vi "Initialize Attributes.vi"(8 "error in (no error)":errorcluster, 10 "Attribute Data":variant, 11 "CS++SimMotor in":refnum<class "CS++SimMotor.lvclass">) -> (0 "error out":errorcluster, 2 "Found?":bool, 3 "CS++SimMotor out":refnum<class "CS++SimMotor.lvclass">)   [LabVIEW 2015, in "CS++SimMotor.lvlib" / "CS++SimMotor.lvclass"]
doc: "Initialize object attribute.\n\nUnique resources should be allocated elsewhere!"
uses:
  CS++SimMotor.lvclass
  CSPP_Core/Classes/CS++ProcessVariables/ProcessVariable/PV.lvclass
  CSPP_Core/Actors/CS++BaseActor/CS++BaseActor.lvclass/CS++BaseActor.ctl
  CSPP_Core/Classes/CS++ProcessVariables/ProcessVariable/PV.lvclass/PV.ctl
  CS++SimMotor.lvclass/CS++SimMotor.ctl
  CSPP_Core/Classes/CS++ProcessVariables/ProcessVariable/Write PV URL.vi
  CSPP_Core/Classes/CS++ProcessVariables/ProcessVariable/Write Type Descriptor.vi
  <vilib>/Utility/error.llb/Error Cluster From Error Code.vi
  CSPP_DeviceBase/CS++Motor/CS++Motor.lvclass
  CSPP_Core/Classes/CS++BaseClasses/Factory/CS++Factory.lvclass
  CSPP_Core/Libraries/Utilities/CS++Utilities.lvlib
  CSPP_Core/Classes/CS++ProcessVariables/CS++ProcessVariables.lvlib
  CSPP_Core/Actors/CS++BaseActor/CS++BaseActor.lvclass
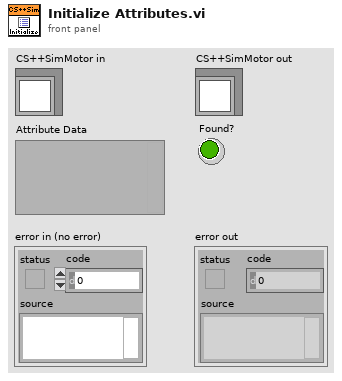
[diagram p1: front panel]
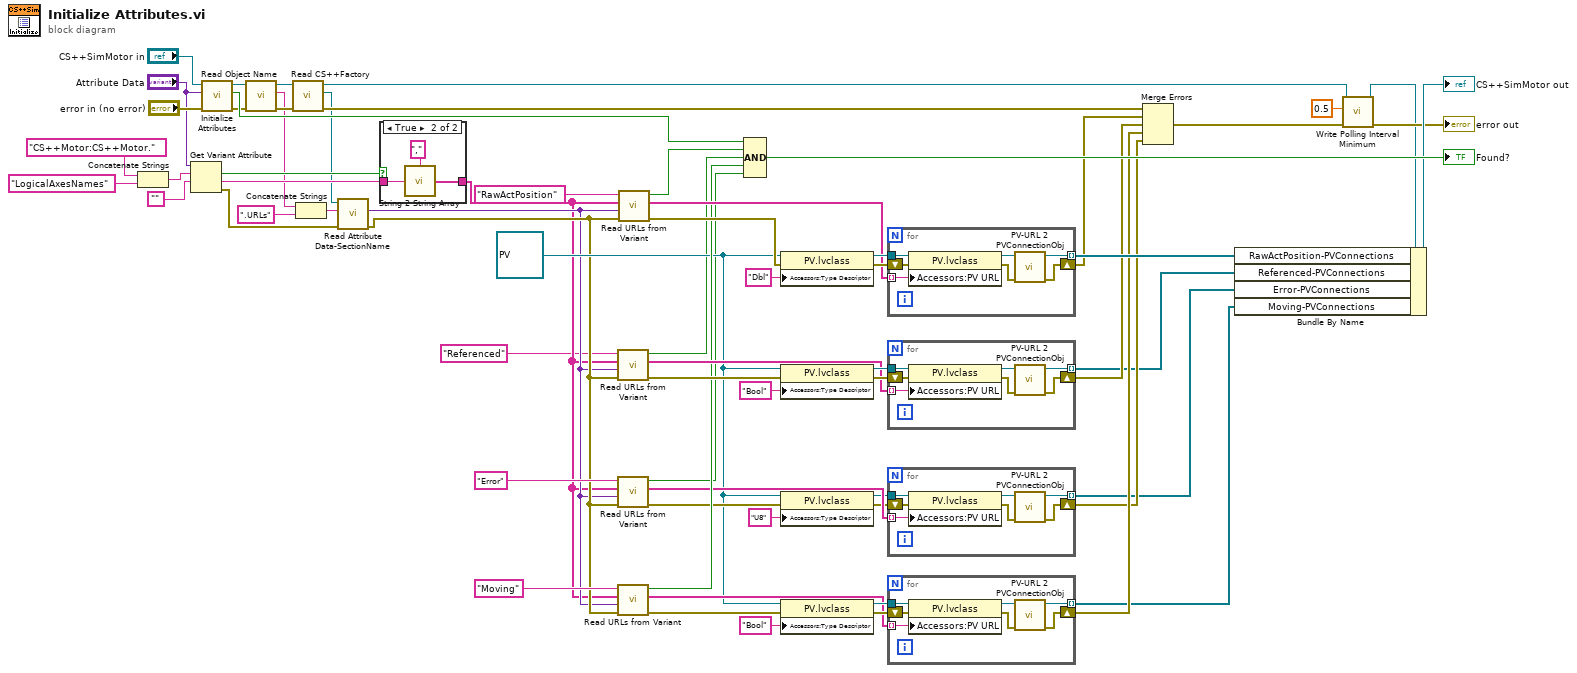
[diagram p0: block diagram]
diagram:
  w16 = refnum<class "PV.lvclass"> refnum ("CS++ProcessVariables.lvlib:PV.lvclass")
  n1 = Concatenate Strings("CS++Motor:CS++Motor.", "LogicalAxesNames" ("string")) -> (w63:string)
  n2 = Get Variant Attribute(Variant="Attribute Data", name=w63, default value (empty Variant)="") -> (found=w59:bool, value=w60:string, error out=w39:errorcluster)  [unwired: 1 in, 1 out]
  n3 = call-parent "Initialize Attributes.vi"("error in (no error)"="error in (no error)", "Attribute Data"="Attribute Data", "CS++Motor in"="CS++SimMotor in") -> ("error out"=w44:errorcluster, "Found?"=w45:bool, "CS++Motor out"=w43:refnum<class "CS++SimMotor.lvclass">)  [unwired: 6 in]
  n4 = call "Read Object Name.vi"("error in (no error)"=w44, "CS++BaseActor in"=w43) -> ("error out"=w46:errorcluster, "Object Name"=w37:string, "CS++BaseActor out"=w47:refnum<class "CS++SimMotor.lvclass">)  [unwired: 7 in]
  n5 = call "Read CS++Factory.vi"("error in (no error)"=w46, "CS++BaseActor in"=w47) -> ("error out"=w42:errorcluster, "CS++Factory"=w38:refnum<class "CS++Factory.lvclass">, "CS++BaseActor out"=w3:refnum<class "CS++SimMotor.lvclass">)  [unwired: 7 in]
  n6 = Concatenate Strings(w37, ".URLs" ("string")) -> (w41:string)
  n7 = call-dynamic "Read Attribute Data-SectionName.vi"("error in (no error)"=w39, "Object Name"=w41, "CS++Factory in"=w38) -> ("error out"=w14:errorcluster, "Attribute Data"=w13:variant)  [unwired: 6 in, 1 out]
  n8 = case shown="True" w59 {
    tunnel: w60 -> [_ w70]
    tunnel: [_ w69] -> w12
    frame False {
    }
    frame True {
      n9 = call "String 2 String Array.vi"("String"=w70, "Delimiter (\",\")"="," ("Delimiter (\",\")")) -> ("Substrings"=w69:string[])
    }
  }
  n10 = call "Read URLs from Variant.vi"("Error In"=w14, "URL Section Data"=w13, "Channel Names"=w12, "URL Prefix"="Referenced") -> ("Error Out"=w35:errorcluster, "URLs"=w32:string[], "Found?"=w9:bool)  [unwired: 4 in, 1 out]
  n11 = call "Read URLs from Variant.vi"("Error In"=w14, "URL Section Data"=w13, "Channel Names"=w12, "URL Prefix"="Error") -> ("Error Out"=w21:errorcluster, "URLs"=w20:string[], "Found?"=w15:bool)  [unwired: 4 in, 1 out]
  n12 = call "Read URLs from Variant.vi"("Error In"=w14, "URL Section Data"=w13, "Channel Names"=w12, "URL Prefix"="Moving") -> ("Error Out"=w26:errorcluster, "URLs"=w27:string[], "Found?"=w25:bool)  [unwired: 4 in, 1 out]
  n13 = call "Read URLs from Variant.vi"("Error In"=w14, "URL Section Data"=w13, "Channel Names"=w12, "URL Prefix"="RawActPosition") -> ("Error Out"=w52:errorcluster, "URLs"=w53:string[], "Found?"=w58:bool)  [unwired: 4 in, 1 out]
  n14 = Compound Arithmetic op=AND(w45, w58, w9, w25, w15) -> (→"Found?":bool)
  n15 = property class="PV.lvclass"(reference=w16, error in=w52, "Accessors:Type Descriptor"="Dbl" ("Type Descriptor")) -> (reference out=w55:refnum<class "PV.lvclass">, error out=w54:errorcluster)
  n16 = property class="PV.lvclass"(reference=w16, error in=w35, "Accessors:Type Descriptor"="Bool" ("Type Descriptor")) -> (reference out=w34:refnum<class "PV.lvclass">, error out=w33:errorcluster)
  n17 = property class="PV.lvclass"(reference=w16, error in=w21, "Accessors:Type Descriptor"="U8" ("Type Descriptor")) -> (reference out=w19:refnum<class "PV.lvclass">, error out=w18:errorcluster)
  n18 = property class="PV.lvclass"(reference=w16, error in=w26, "Accessors:Type Descriptor"="Bool" ("Type Descriptor")) -> (reference out=w28:refnum<class "PV.lvclass">, error out=w29:errorcluster)
  n19 = for {
    tunnel: w55 -> [w76]
    tunnel: w53 -> [w75] mode=indexing
    tunnel: [w74] -> w49 mode=indexing
    shift-right: [w73] -> w48
    shift-left: w54 -> [w71]
    n20 = property class="PV.lvclass"(reference=w76, error in=w71, "Accessors:PV URL"=w75) -> (reference out=w77:refnum<class "PV.lvclass">, error out=w72:errorcluster)
    n21 = call "PV-URL 2 PVConnectionObj.vi"("Error In"=w72, "PV"=w77) -> ("Error Out"=w73:errorcluster, "PVConnection"=w74:refnum<class "PVConnection.lvclass">)  [unwired: 7 in, 1 out]
  }
  n22 = for {
    tunnel: w34 -> [w83]
    tunnel: w32 -> [w82] mode=indexing
    tunnel: [w81] -> w7 mode=indexing
    shift-right: [w80] -> w31
    shift-left: w33 -> [w78]
    n23 = property class="PV.lvclass"(reference=w83, error in=w78, "Accessors:PV URL"=w82) -> (reference out=w84:refnum<class "PV.lvclass">, error out=w79:errorcluster)
    n24 = call "PV-URL 2 PVConnectionObj.vi"("Error In"=w79, "PV"=w84) -> ("Error Out"=w80:errorcluster, "PVConnection"=w81:refnum<class "PVConnection.lvclass">)  [unwired: 7 in, 1 out]
  }
  n25 = for {
    tunnel: w19 -> [w90]
    tunnel: w20 -> [w89] mode=indexing
    tunnel: [w88] -> w6 mode=indexing
    shift-right: [w87] -> w11
    shift-left: w18 -> [w85]
    n26 = property class="PV.lvclass"(reference=w90, error in=w85, "Accessors:PV URL"=w89) -> (reference out=w91:refnum<class "PV.lvclass">, error out=w86:errorcluster)
    n27 = call "PV-URL 2 PVConnectionObj.vi"("Error In"=w86, "PV"=w91) -> ("Error Out"=w87:errorcluster, "PVConnection"=w88:refnum<class "PVConnection.lvclass">)  [unwired: 7 in, 1 out]
  }
  n28 = for {
    tunnel: w28 -> [w97]
    tunnel: w27 -> [w96] mode=indexing
    tunnel: [w95] -> w8 mode=indexing
    shift-right: [w94] -> w23
    shift-left: w29 -> [w92]
    n29 = property class="PV.lvclass"(reference=w97, error in=w92, "Accessors:PV URL"=w96) -> (reference out=w98:refnum<class "PV.lvclass">, error out=w93:errorcluster)
    n30 = call "PV-URL 2 PVConnectionObj.vi"("Error In"=w93, "PV"=w98) -> ("Error Out"=w94:errorcluster, "PVConnection"=w95:refnum<class "PVConnection.lvclass">)  [unwired: 7 in, 1 out]
  }
  n31 = Merge Errors(w42, w48, w31, w23, w11) -> (w5:errorcluster)
  n32 = call "Write Polling Interval Minimum.vi"("error in (no error)"=w5, "Polling Interval Minimum"=dbl[unit] 0.5, "CS++BaseActor in"=w3) -> ("error out"=→"error out":errorcluster, "CS++BaseActor out"=w2:refnum<class "CS++SimMotor.lvclass">)  [unwired: 7 in]
  n33 = Bundle By Name(cluster=w2, "RawActPosition-PVConnections"=w49, "Referenced-PVConnections"=w7, "Error-PVConnections"=w6, "Moving-PVConnections"=w8) -> (→"CS++SimMotor out":refnum<class "CS++SimMotor.lvclass">)
